vi "T7_Write_FLOAT32_Register.vi"(7 "FLOAT32 to Write":sgl=1.23, 9 "LabJack TestFLOAT32 Register":i32=55124, 10 "Remote Port":u16=502, 11 "Remote IP Address":string="192.168.1.15") -> ()   [LabVIEW 2017]
panel:
  # "MB Ethernet Example Master.vi\n\nInstructions\n1.Use Kipling to find your devices IP address & modify the\n\"Remote IP Addres\"\n2. Run this VI\n3. Change value of \"FLOAT32 to Write\" & press \"Write Data\""
  # "TCP Parameters"
  # "Test Write & Read of TEST_UINT32 Register"
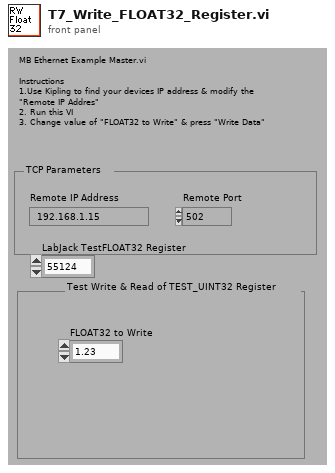
[diagram p1: front panel]
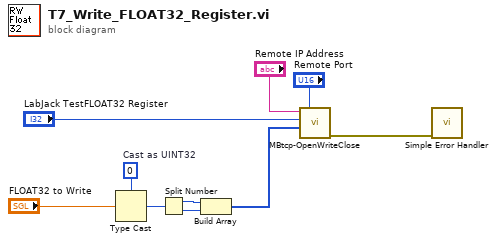
[diagram p0: block diagram]
diagram:
  w9 = u32 0  # Cast as UINT32
  n1 = Type Cast(type=w9, x="FLOAT32 to Write") -> (*(type *) &x=w8:u32)
  n2 = Split Number(x=w8) -> (hi(x)=w7:u16, lo(x)=w6:u16)
  n3 = Build Array(w7, w6) -> (w2:u16[])
  n4 = call "MBtcp-OpenWriteClose.vi"("Port"="Remote Port", "Values"=w2, "RegisterAddr"="LabJack TestFLOAT32 Register", "IP Address"="Remote IP Address") -> ("error out"=w1:errorcluster)  [unwired: 7 in]
  n5 = call <vilib>:"Simple Error Handler.vi"("error in (no error)"=w1) -> ()  [unwired: 1 in, 8 out]
